vi "IniDisplay.vi"(8 "error in (no error)":errorcluster caption="错误输入（无错误）", 10 "通道选择":string[](array[string]), 11 "DigitalDisplay 输入":refnum<class "DigitalDisplay.lvclass">) -> (0 "error out":errorcluster caption="错误输出", 3 "DigitalDisplay 输出":refnum<class "DigitalDisplay.lvclass">)   [LabVIEW 2018, in "DataDisplay.lvlib" / "DigitalDisplay.lvclass"]
uses:
  DigitalDisplay.lvclass
  <vilib>/Utility/miscctls.llb/LVPointTypeDef.ctl
  DigitalDisplay.lvclass/DigitalDisplay.ctl
  SubVI/DD_Parameter.vi
  DataDisplay.lvlib
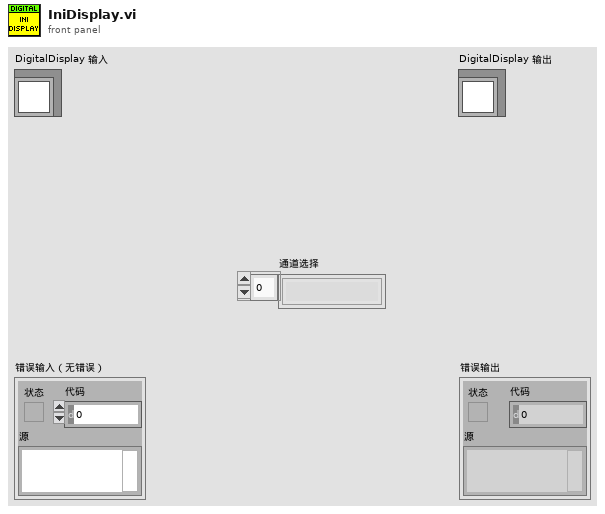
[diagram p1: front panel]
types:
  T1 = typedef "LVPointTypeDef.ctl" = cluster{"Horizontal":i16, "Vertical":i16}
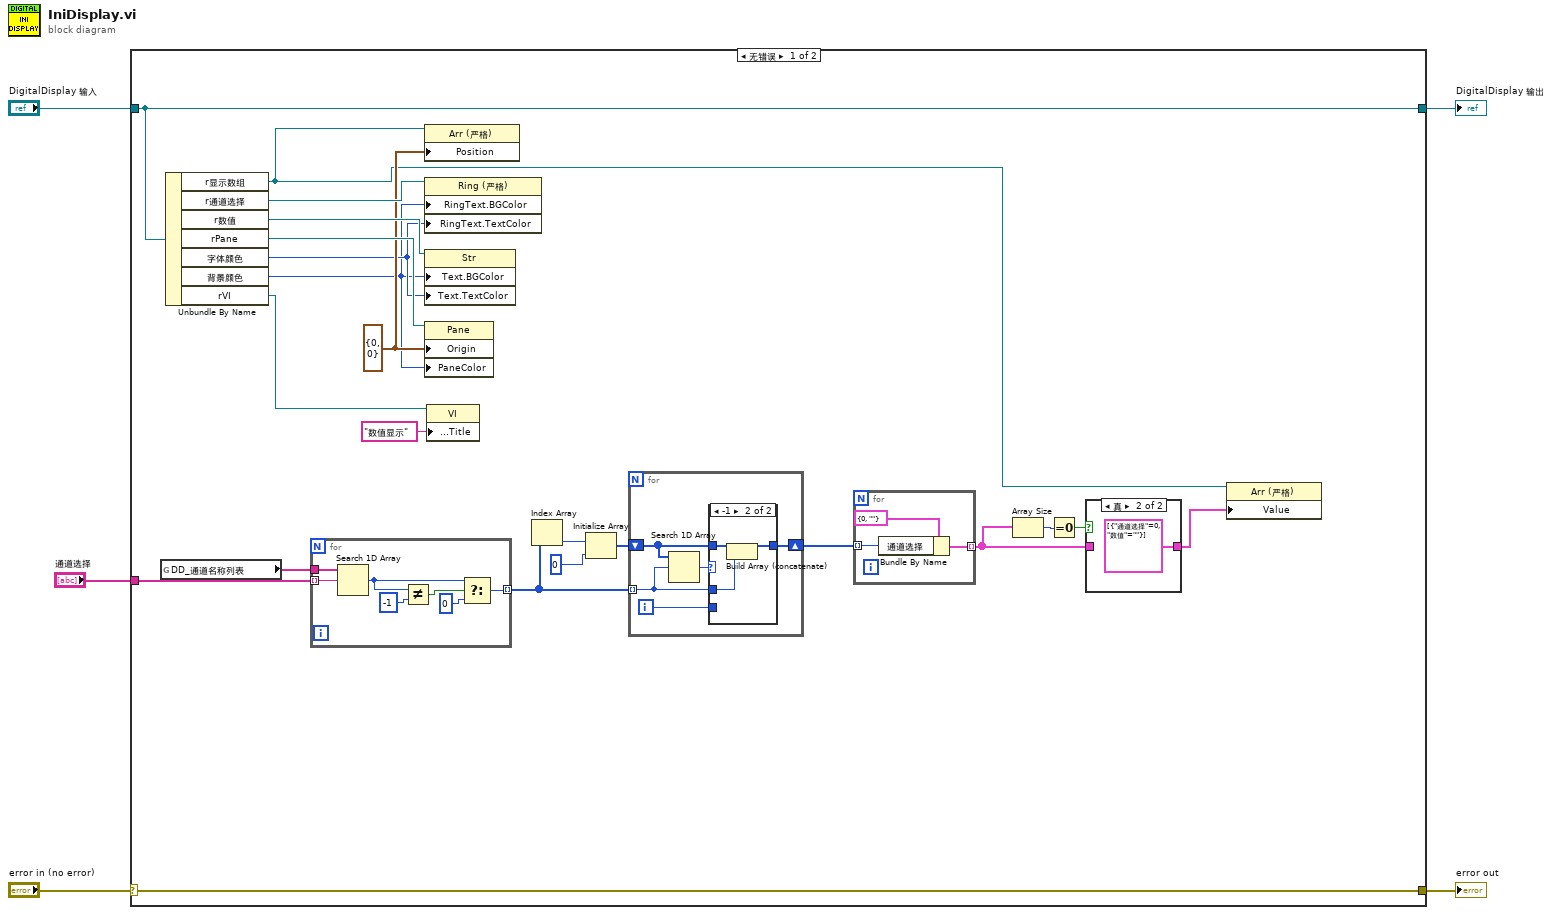
[diagram p0: block diagram]
diagram:
  n1 = case shown="无错误" "error in (no error)" {
    selector: "error in (no error)" -> [w27 w50]
    tunnel: [w27 w50] -> w4
    tunnel: [w26 w49] -> w2
    tunnel: "DigitalDisplay 输入" -> [w26 w49]
    tunnel: "通道选择" -> [w16 _]
    frame No Error {
      w22 = T1 {"Horizontal"=0, "Vertical"=0} ("原点")
      n2 = global read "DD_Parameter.vi" "DD_通道名称列表"() -> (w17:string[])
      n3 = Unbundle By Name(w26) -> ("r显示数组"=w10:refnum<vi>, "r通道选择"=w24:refnum<vi>, "r数值"=w23:refnum<vi>, "rPane"=w25:refnum<vi>, "字体颜色"=w21:u32, "背景颜色"=w20:u32, "rVI"=w19:refnum<vi>)
      n4 = for {
        tunnel: w17 -> [w48]
        tunnel: w16 -> [w43] mode=indexing
        tunnel: [w42] -> w12 mode=indexing
        n5 = Search 1D Array(1D array=w48, element=w43) -> (index of element=w45:i32)  [unwired: 1 in]
        n6 = Not Equal?(x=w45, y=-1) -> (x != y?=w46:bool)
        n7 = Select(t=w45, s=w46, f=0) -> (s? t:f=w42:i32)
      }
      n8 = property class="Arr (严格)"(reference=w10, "Position"=w22) -> ()  [unwired: 1 in, 2 out]
      n9 = property class="Ring (严格)"(reference=w24, "RingText.BGColor"=w20, "RingText.TextColor"=w21) -> ()  [unwired: 1 in, 2 out]
      n10 = property class="Str"(reference=w23, "Text.BGColor"=w20, "Text.TextColor"=w21) -> ()  [unwired: 1 in, 2 out]
      n11 = property class="Pane"(reference=w25, "Origin"=w22, "PaneColor"=w20) -> ()  [unwired: 1 in, 2 out]
      n12 = property class="VI"(reference=w19, "Front Panel.Title"="数值显示" ("前面板窗口:标题")) -> ()  [unwired: 1 in, 2 out]
      n13 = Index Array(array=w12) -> (element=w15:i32)  [unwired: 1 in]
      n14 = Initialize Array(w15, 0 ("Dimension Size")) -> (w14:i32[])
      n15 = for {
        tunnel: w12 -> [w36] mode=indexing
        shift-right: [w35] -> w11
        shift-left: w14 -> [w34]
        i -> [w33]
        n16 = Search 1D Array(1D array=w34, element=w36) -> (index of element=w37:i32)  [unwired: 1 in]
        n17 = case shown="-1" w37 {
          tunnel: w36 -> [_ w41]
          tunnel: [w38 w39] -> w35
          tunnel: w34 -> [w38 w40]
          tunnel: w33 -> [_ _]
          frame Default {
          }
          frame -1 {
            n18 = Build Array (concatenate)(w40, w41) -> (w39:i32[])
          }
        }
      }
      n19 = for {
        tunnel: w11 -> [w31] mode=indexing
        tunnel: [w30] -> w6 mode=indexing
        n20 = Bundle By Name(cluster=cluster{"通道选择":u16, "数值":string} {"通道选择"=0, "数值"=""} ("簇"), "通道选择"=w31) -> (w30:cluster{"通道选择":u16, "数值":string})
      }
      n21 = Array Size(array=w6) -> (size(s)=w9:i32)
      n22 = Equal To 0?(x=w9) -> (x = 0?=w8:bool)
      n23 = case shown="真" w8 {
        tunnel: [w28 cluster{"通道选择":u16, "数值":string}[] [{"通道选择"=0, "数值"=""}] ("添加的数组")] -> w7
        tunnel: w6 -> [w28 _]
        frame False {
        }
        frame True {
        }
      }
      n24 = property class="Arr (严格)"(reference=w10, "Value"=w7) -> ()  [unwired: 1 in, 2 out]
    }
    frame Error {
    }
  }
  "error out" <- w4
  "DigitalDisplay 输出" <- w2
